vi "niRFUtil MT UTIL Filter Taps - Full Raised Cosine.vi"(0 "Samples Per Symbol (16)":i32=16, 5 "Filter Length (3)":i32=3, 7 "Alpha (0.5)":dbl=0.5 format="%.2f", 11 "error in (no error)":errorcluster) -> (4 "Filter Coefficients":T1 min=0 max=127 format="%.2f", 15 "error out":errorcluster)   [LabVIEW 2015, in "niRFUtil.lvlib"]
uses:
  niRFUtil.lvlib
  Includes/niRFUtil INC Real Array.ctl
panel:
  out "Full Raised Cosine":sgl[](graph)
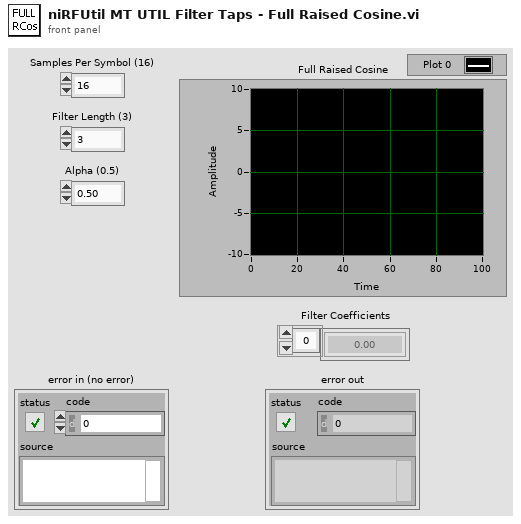
[diagram p1: front panel]
types:
  T1 = typedef "niRFUtil.lvlib/niRFUtil INC Real Array.ctl" = sgl[]
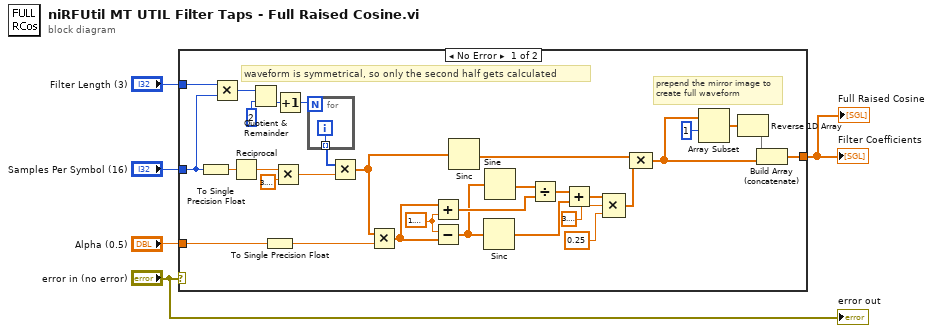
[diagram p0: block diagram]
diagram:
  n1 = case shown="No Error" "error in (no error)" {
    tunnel: "Filter Length (3)" -> [w30 _]
    tunnel: "Samples Per Symbol (16)" -> [w7 _]
    tunnel: "Alpha (0.5)" -> [w12 _]
    tunnel: [w9 _] -> w2
    frame No Error {
      w28 = sgl 1.5707964
      # "prepend the mirror image to create full waveform"
      # "waveform is symmetrical, so only the second half gets calculated"
      n2 = To Single Precision Float(number=w7) -> (single precision float=w8:sgl)
      n3 = Multiply(x=w30, y=w7) -> (x*y=w36:i32)
      n4 = Reciprocal(x=w8) -> (1/x=w29:sgl)
      n5 = Quotient & Remainder(x=w36, y=2) -> (floor(x/y)=w33:i32)  [unwired: 1 out]
      n6 = To Single Precision Float(number=w12) -> (single precision float=w6:sgl)
      n7 = Multiply(x=w29, y=sgl 3.1415927) -> (x*y=w14:sgl)
      n8 = Increment(x=w33) -> (x+1=w34:i32)
      n9 = for {
        N: w34 -> [_]
        tunnel: [w37] -> w15 mode=indexing
        i -> [w37]
      }
      n10 = Multiply(x=w15, y=w14) -> (x*y=w13:sgl[])
      n11 = Multiply(x=w13, y=w6) -> (x*y=w16:sgl[])
      n12 = Add(x=w16, y=w28) -> (x+y=w11:sgl[])
      n13 = Subtract(x=w28, y=w16) -> (x-y=w10:sgl[])
      n14 = Sinc(1:w13) -> (0:w31:sgl[])
      n15 = Sinc(1:w10) -> (0:w25:sgl[])
      n16 = Sine(x=w10) -> (sin(x)=w27:sgl[])
      n17 = Divide(x=w27, y=w11) -> (x/y=w26:sgl[])
      n18 = Add(x=w26, y=w25) -> (x+y=w24:sgl[])
      n19 = Compound Arithmetic op=MULTIPLY(w24, sgl 3.1415927, sgl 0.25) -> (w23:sgl[])
      n20 = Compound Arithmetic op=MULTIPLY(w31, w23) -> (w18:sgl[])
      n21 = Array Subset(array=w18, index=1 ("Array Index")) -> (w20:sgl[])  [unwired: 1 in]
      n22 = Reverse 1D Array(array=w20) -> (reversed array=w19:sgl[])
      n23 = Build Array (concatenate)(w19, w18) -> (w9:sgl[])
    }
    frame Error {
    }
  }
  "Full Raised Cosine" <- w2
  "Filter Coefficients" <- w2
  "error out" <- "error in (no error)"
